vi "Read Channel URL list.vi"(8 "error in":errorcluster, 11 "CVT editor node in":refnum<class "TEC editor node.lvclass">) -> (0 "error out":errorcluster, 2 "URLs":string[](array[string]), 3 "CVT editor node out":refnum<class "TEC editor node.lvclass">)   [LabVIEW 2013, in "TEC editor node.lvclass"]
uses:
  TEC editor node.lvclass
  <vilib>/NI/Tag Bus Data Framework/Configuration Editor/Classes/Module editor node/module editor node.lvclass
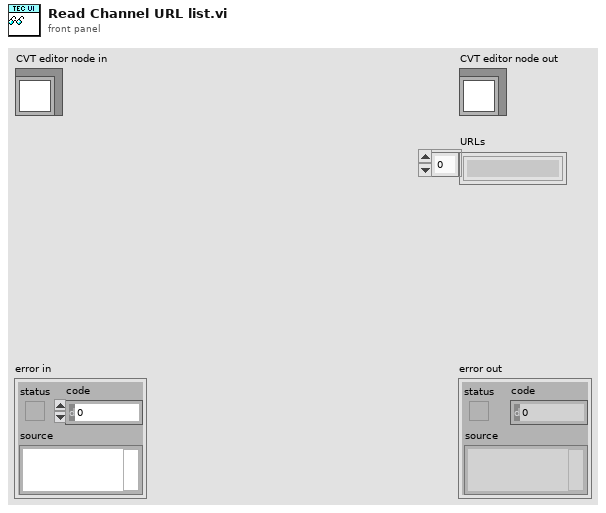
[diagram p1: front panel]
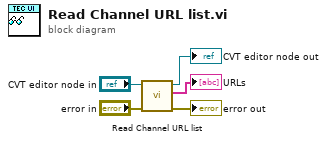
[diagram p0: block diagram]
diagram:
  n1 = call-parent "Read Channel URL list.vi"("error in"="error in", "Module Editor Node in"="CVT editor node in") -> ("error out"=→"error out":errorcluster, "URLs"=→"URLs":string[], "Module Editor Node out"=→"CVT editor node out":refnum<class "TEC editor node.lvclass">)  [unwired: 7 in]
